vi "Multiple Element Enqueue - Main Loop.vi"(7 "Enqueue to (Back of Queue)":enum16{"Back of Queue", "Front of Queue"}(ring), 8 "error in (no error)":errorcluster, 10 "Elements to enqueue (Array)":T1[](array[typedef]), 11 "Queue In":refnum<queue>) -> (0 "error out":errorcluster, 3 "QueueOut":refnum<queue>)   [LabVIEW 2019]
uses:
  Type Definitions/Main Loop Queue Data.ctl
  Type Definitions/Main Loop States.ctl
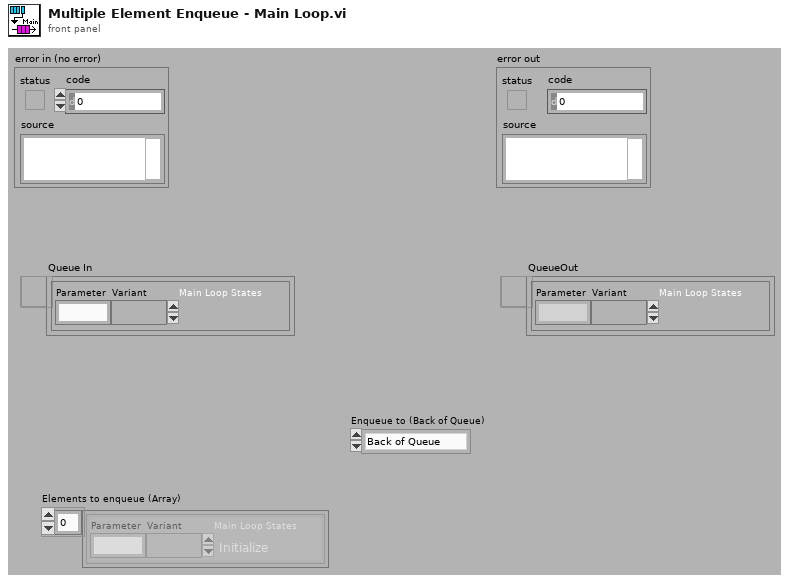
[diagram p1: front panel]
types:
  T1 = typedef "Main Loop Queue Data.ctl" = cluster{"Parameter":string, "Variant":variant, "Main Loop States":T2}
  T2 = typedef "Main Loop States.ctl" = enum16{"  -----  Core  -----  ", "Blank", "Idle", "Initialize", "Shutdown", "Error", "  ----- meerstetter TEC Functions -----  ", "TE Controller"}
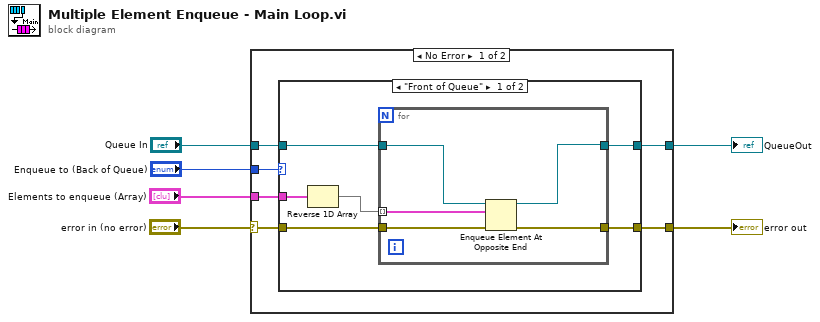
[diagram p0: block diagram]
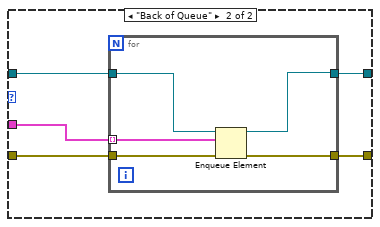
[diagram p2: hidden frame]
diagram:
  n1 = case shown="No Error" "error in (no error)" {
    selector: "error in (no error)" -> [w10 w34]
    tunnel: [w12 w34] -> w6
    tunnel: [w11 _] -> w4
    tunnel: "Queue In" -> [w9 _]
    tunnel: "Elements to enqueue (Array)" -> [w8 _]
    tunnel: "Enqueue to (Back of Queue)" -> [w7 _]
    frame No Error {
      n2 = case shown="\"Front of Queue\"" w7 {
        tunnel: [w18 w28] -> w12
        tunnel: [w17 w27] -> w11
        tunnel: w10 -> [w16 w26]
        tunnel: w9 -> [w15 w25]
        tunnel: w8 -> [w14 w24]
        frame "Front of Queue" {
          n3 = Reverse 1D Array(array=w14) -> (reversed array=w13:T1[])
          n4 = for {
            tunnel: w16 -> [w23]
            tunnel: w13 -> [w22] mode=indexing
            tunnel: [w21] -> w18
            tunnel: [w20] -> w17
            tunnel: w15 -> [w19]
            n5 = Enqueue Element At Opposite End(queue=w19, element=w22, error in (no error)=w23) -> (queue out=w20:refnum<queue>, error out=w21:errorcluster)  [unwired: 1 in, 1 out]
          }
        }
        frame "Back of Queue" {
          n6 = for {
            tunnel: w26 -> [w33]
            tunnel: w24 -> [w32] mode=indexing
            tunnel: [w31] -> w28
            tunnel: [w30] -> w27
            tunnel: w25 -> [w29]
            n7 = Enqueue Element(queue=w29, element=w32, error in (no error)=w33) -> (queue out=w30:refnum<queue>, error out=w31:errorcluster)  [unwired: 1 in, 1 out]
          }
        }
      }
    }
    frame Error {
    }
  }
  "error out" <- w6
  "QueueOut" <- w4
